vi "(SubVI)File Gen_Get File Path.vi"(6 "Common?":bool, 7 "Use Timestamp":bool, 8 "error in (no error)":errorcluster caption="에러 입력(에러 없음)", 9 "File Extension (.txt)":string=".txt", 10 "File Name":string, 11 "Folder Name":string) -> (0 "error out":errorcluster caption="에러 출력", 2 "file or folder exists?":bool caption="exist?", 3 "Path":path)   [LabVIEW 2020]
panel:
  # "(SubVI)File Gen_Get File Path.vi By hspark\n\nDescription : 폴더와 파일 이름, 확장자 명을 입력 받아 경로를 생성하는 VI\n\nInput : \n1. Folder Name : Default Path에 생성될 폴더 이름\n2. File Name : 생성할 파일 이름\n3. File Extension (.txt) : 파일 확장자명. 기본 값은 '.txt' 이며 '.'의 포함 여부는 상관 없음\n4. Use Timestamp : True 입력 시 현재 시간을 파일명 앞에 입력함\n                           형식 : YYYYmmdd_HHMMSS_File name\n2. Common? : false 입력 시 data 폴더 안에 Chip Type 폴더 사용\n\nOutput : \n1. Path : 생성된 경로. 폴더는 생성되나, 파일은 생성되지 않음\n2. exist? : 이미 같은 경로의 파일이 있는 경우 True 출력\n\nLabVIEW Version : 2020 SP1 이상\n\nNote :\n파일 이름에서 '\\', ':', '/' 등 Windows에서 경로에 사용할 수 없는 문자는 제거됨 (폴더 이름에 대해서는 수행하지 않음)\n파일 이름에서 사용할 수 없는 문자를 제거한 후 빈 문자열인 경우 현재 시간을 파일명으로 사용함\n\nUpdate : 2022.02.08"
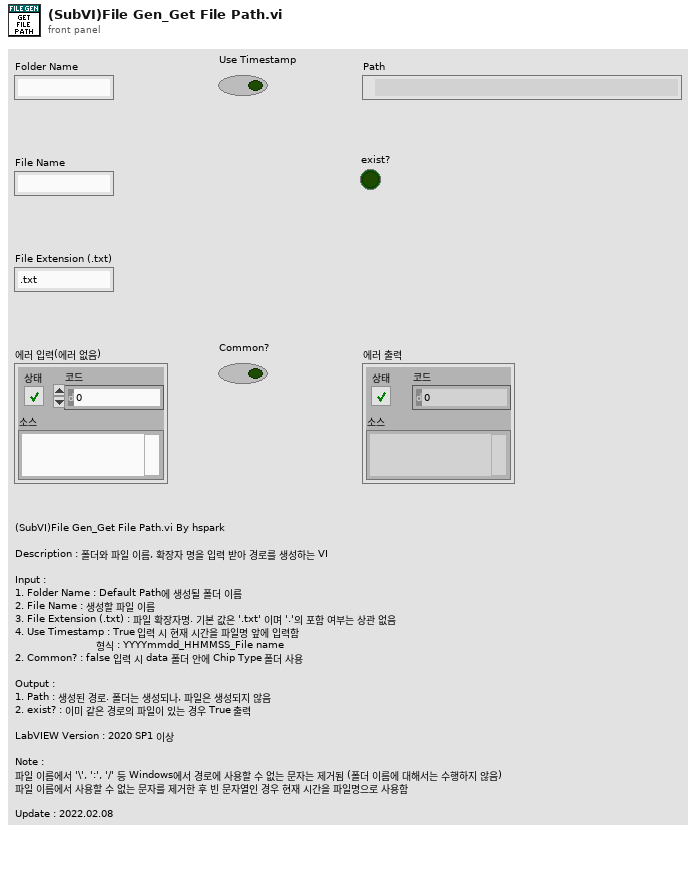
[diagram p1: front panel]
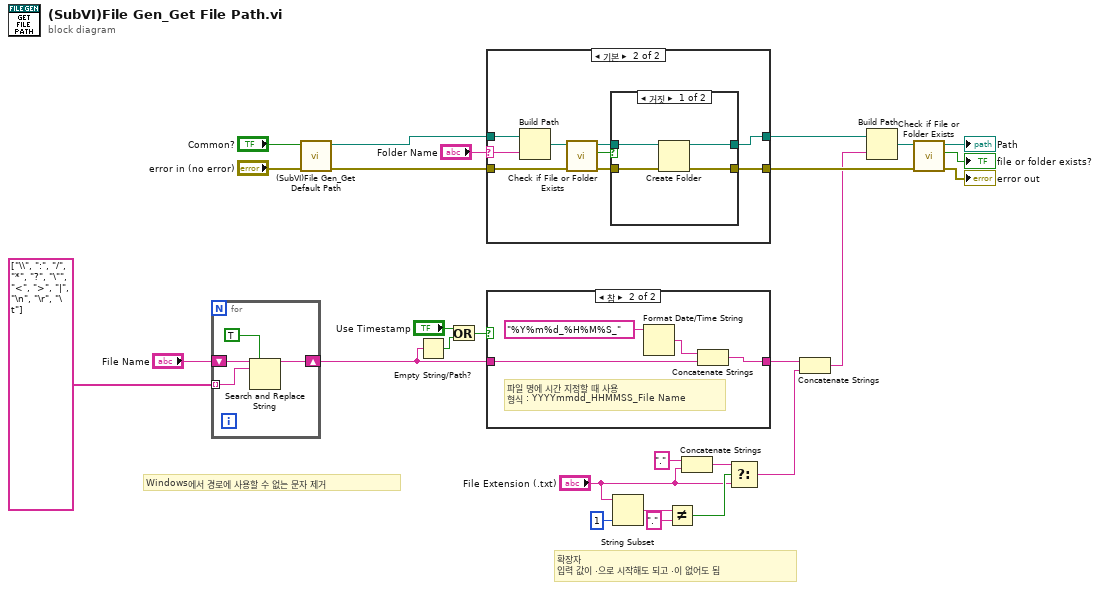
[diagram p0: block diagram]
diagram:
  # "확장자\n입력 값이 .으로 시작해도 되고 .이 없어도 됨"
  # "Windows에서 경로에 사용할 수 없는 문자 제거"
  n1 = for {
    tunnel: string[] ["\\", ":", "/", "*", "?", "\"", "<", ">", "|", "\n", "\r", "\t"] -> [w30] mode=indexing
    shift-right: [w29] -> w3
    shift-left: "File Name" -> [w31]
    n2 = Search and Replace String(replace all?=TRUE ("모두 대체? (거짓)"), input string=w31, search string=w30) -> (result string=w29:string)  [unwired: 5 in, 3 out]
  }
  n3 = call "(SubVI)File Gen_Get Default Path.vi"("error in (no error)"="error in (no error)", "Common?"="Common?") -> ("error out"=w25:errorcluster, "default path"=w27:path)  [unwired: 8 in]
  n4 = Empty String/Path?(string/path=w3) -> (empty?=w1:bool)
  n5 = Or(x="Use Timestamp", y=w1) -> (x .or. y?=w2:bool)
  n6 = case shown="기본" "Folder Name" {
    selector: "Folder Name" -> [_ w41]
    tunnel: w27 -> [w33 w42]
    tunnel: [w33 w35] -> w22
    tunnel: w25 -> [w32 w36]
    tunnel: [w32 w34] -> w21
    frame "" {
      # "폴더 명 입력이 없을 경우\nDefault Path로 함"
    }
    frame Default {
      n7 = Build Path(base path=w42, name or relative path=w41) -> (appended path=w40:path)
      n8 = call <vilib>:"Check if File or Folder Exists.vi"("error in (no error)"=w36, "path"=w40) -> ("error out"=w37:errorcluster, "file or folder exists?"=w39:bool, "dup path"=w38:path)  [unwired: 7 in]
      n9 = case shown="거짓" w39 {
        tunnel: w38 -> [w44 w48]
        tunnel: w37 -> [w46 w47]
        tunnel: [w43 w48] -> w35
        tunnel: [w45 w47] -> w34
        frame False {
          n10 = Create Folder(path (use dialog)=w44, error in=w46) -> (created path=w43:path, error out=w45:errorcluster)  [unwired: 1 in, 1 out]
        }
        frame True {
        }
      }
    }
  }
  n11 = case shown="참" w2 {
    tunnel: w3 -> [w49 w52]
    tunnel: [w49 w51] -> w16
    frame False {
    }
    frame True {
      # "파일 명에 시간 지정할 때 사용\n형식 : YYYYmmdd_HHMMSS_File Name"
      n12 = Format Date/Time String(time format string (%c)="%Y%m%d_%H%M%S_" ("시간 포맷 문자열 (%c)")) -> (date/time string=w50:string)  [unwired: 2 in]
      n13 = Concatenate Strings(w50, w52) -> (w51:string)
    }
  }
  n14 = String Subset(string="File Extension (.txt)", length (rest)=1 ("길이(나머지)")) -> (substring=w13:string)  [unwired: 1 in]
  n15 = Not Equal?(x=w13, y=".") -> (x != y?=w11:bool)
  n16 = Concatenate Strings("." ("문자열"), "File Extension (.txt)") -> (w10:string)
  n17 = Select(t=w10, s=w11, f="File Extension (.txt)") -> (s? t:f=w7:string)
  n18 = Concatenate Strings(w16, w7) -> (w15:string)
  n19 = Build Path(base path=w22, name or relative path=w15) -> (appended path=w23:path)
  n20 = call <vilib>:"Check if File or Folder Exists.vi"("error in (no error)"=w21, "path"=w23) -> ("error out"=→"error out":errorcluster, "file or folder exists?"=→"file or folder exists?":bool, "dup path"=→"Path":path)  [unwired: 7 in]
